vi "setValue.vi"(8 "error in (no error)":errorcluster, 10 "Value":dbl, 11 "tBSONDouble in":refnum<class "tBSONDouble.lvclass">) -> (0 "error out":errorcluster, 3 "tBSONDouble out":refnum<class "tBSONDouble.lvclass">)   [LabVIEW 2013, in "BSON.lvlib" / "tBSONDouble.lvclass"]
uses:
  tBSONDouble.lvclass
  tBSONDouble.lvclass/tBSONDouble.ctl
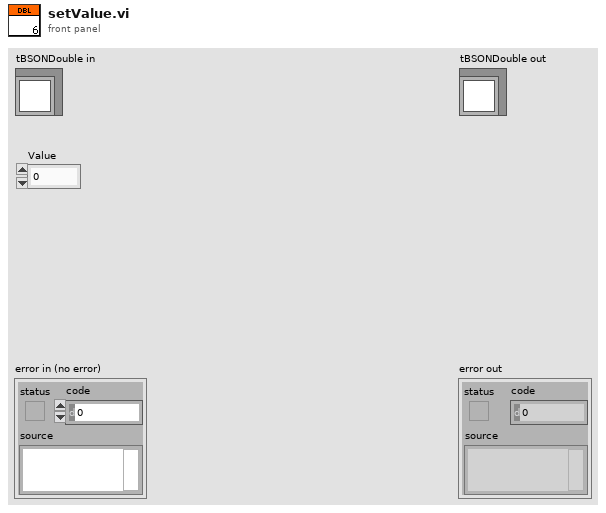
[diagram p1: front panel]
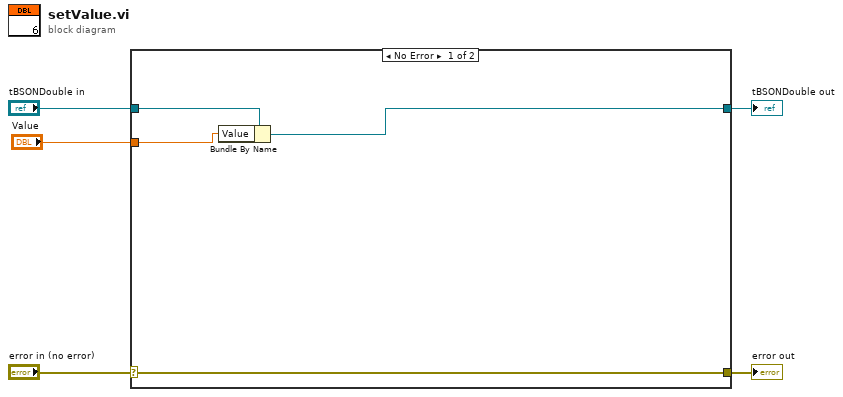
[diagram p0: block diagram]
diagram:
  n1 = case shown="No Error" "error in (no error)" {
    selector: "error in (no error)" -> [w9 w11]
    tunnel: [w9 w11] -> w4
    tunnel: [w6 w10] -> w2
    tunnel: "tBSONDouble in" -> [w7 w10]
    tunnel: "Value" -> [w8 _]
    frame No Error {
      n2 = Bundle By Name(cluster=w7, "Value"=w8) -> (w6:refnum<class "tBSONDouble.lvclass">)
    }
    frame Error {
    }
  }
  "error out" <- w4
  "tBSONDouble out" <- w2
